vi "setFPGA.vi"(10 "FPGA":refnum<class "FPGA.lvclass">, 11 "OuterLoopClockIRQ in":refnum<class "OuterLoopClockIRQ.lvclass">) -> (3 "OuterLoopClockIRQ out":refnum<class "OuterLoopClockIRQ.lvclass">)   [LabVIEW 2016, in "OuterLoopClockIRQ.lvclass"]
uses:
  OuterLoopClockIRQ.lvclass
  FPGA/FPGA.lvclass
  OuterLoopClockIRQ.lvclass/OuterLoopClockIRQ.ctl
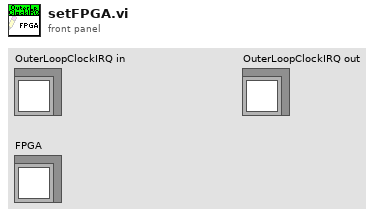
[diagram p1: front panel]
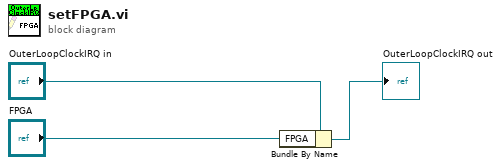
[diagram p0: block diagram]
diagram:
  n1 = Bundle By Name(cluster="OuterLoopClockIRQ in", "FPGA"="FPGA") -> (→"OuterLoopClockIRQ out":refnum<class "OuterLoopClockIRQ.lvclass">)
